vi "Get Epsilon Current.vi"(11 "AnytimeDStar in":refnum<class "NI_Robotics_AnytimeDStar.lvclass">) -> (2 "epsilon current":dbl, 3 "AnytimeDStar out":refnum<class "NI_Robotics_AnytimeDStar.lvclass">)   [LabVIEW 2017, in "NI_Robotics_AnytimeDStar.lvclass"]
uses:
  <vilib>/robotics/Navigation/Anytime D Star/NI_Robotics_AnytimeDStar.lvclass
  <vilib>/robotics/Navigation/Anytime D Star/NI_Robotics_AnytimeDStar.lvclass/NI_Robotics_AnytimeDStar.ctl
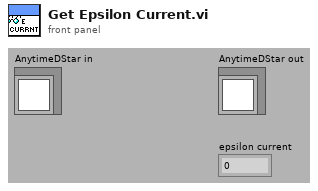
[diagram p1: front panel]
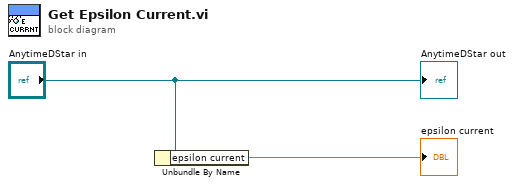
[diagram p0: block diagram]
diagram:
  n1 = Unbundle By Name("AnytimeDStar in") -> ("epsilon current"=→"epsilon current":dbl)
  "AnytimeDStar out" <- "AnytimeDStar in"
